vi "Create Global MetaData Channel_ex.vi"() -> ()   [LabVIEW 2019]
uses:
  <vilib>/NI VeriStand/Custom Device API/Custom Device Item Ref.ctl
  Control 10.ctl
  Scripting API/Polymorphic/Create Channel/Create Global Command Single Channel_Format.vi
  Scripting API/Scripting API.lvlib
  <vilib>/NI VeriStand/Custom Device API/Custom Device API.lvlib
panel:
  out "Instrument Addon Refnum Out":T1=18446744073709551615 format="%.0x"
  out "Channel Refnum":T1=18446744073709551615 format="%.0x"
  out "Error Out":errorcluster
  in  "Instrument Addon Refnum In":T1=18446744073709551615 format="%.0x"
  in  "Error In":errorcluster
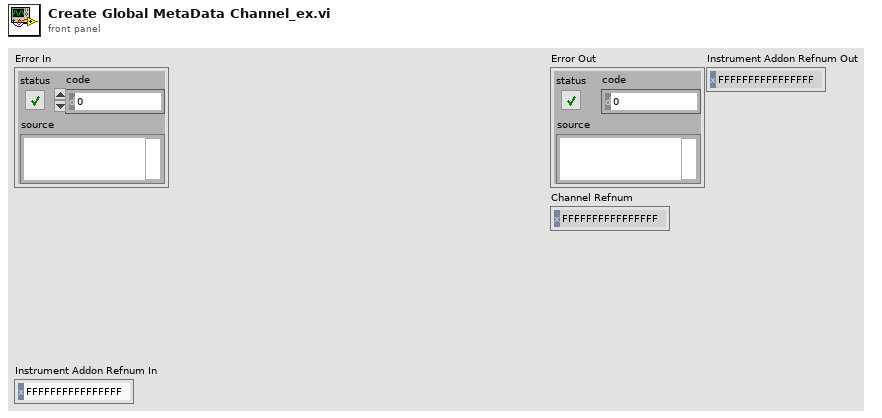
[diagram p1: front panel]
types:
  T1 = typedef "Custom Device API.lvlib/Custom Device Item Ref.ctl" = u64
  T2 = typedef "Control 10.ctl" = cluster{"Format String":string, "Default Value":dbl, "Units":string}
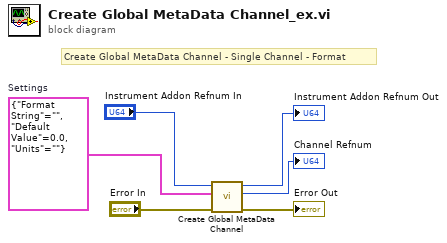
[diagram p0: block diagram]
diagram:
  w1 = T2 {"Format String"="", "Default Value"=0.0, "Units"=""}  # Settings
  # "Create Global MetaData Channel - Single Channel - Format"
  n1 = call-poly "Create Global MetaData Channel.vi"("Error In"="Error In", "Settings"=w1, "Instrument Addon Refnum In"="Instrument Addon Refnum In") -> ("Error Out"=→"Error Out":errorcluster, "Channel Refnum"=→"Channel Refnum":T1, "Instrument Addon Refnum Out"=→"Instrument Addon Refnum Out":T1)  [unwired: 6 in]
